vi "DSF.Engine.Framework.Create.vi"(8 "error in (no error)":errorcluster, 9 "Framework Configuration":refnum<class "DSF.Shared.Configuration.Framework.lvclass">, 10 "Framework Runtime":refnum<class "DSF.Engine.Runtime.Framework.lvclass">, 11 "Framework type":refnum<class "Framework.lvclass">) -> (0 "error out":errorcluster, 3 "Framework":refnum<class "Framework.lvclass">)   [LabVIEW 2016, in "DSF.Engine.lvlib" / "Framework.lvclass"]
uses:
  Framework.lvclass
  DSF.Engine.Runtime.Framework.lvclass
  Shared/Classes/Framework/DSF.Shared.Configuration.Framework.lvclass
  Framework.lvclass/Framework.ctl
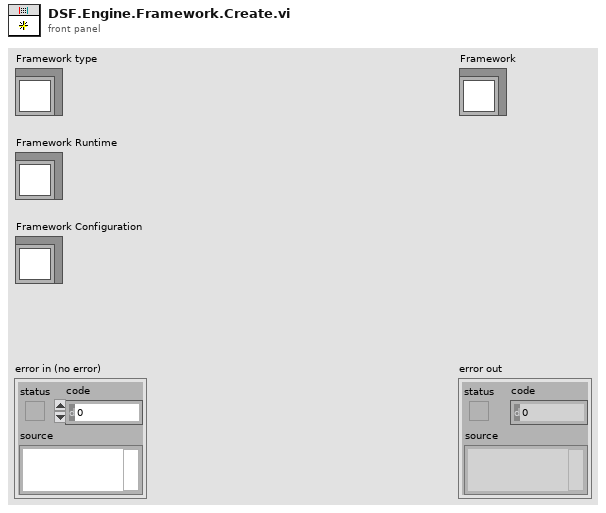
[diagram p1: front panel]
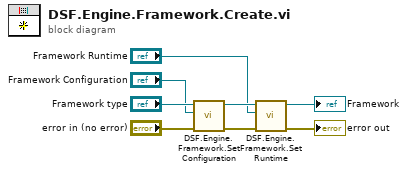
[diagram p0: block diagram]
diagram:
  n1 = call "DSF.Engine.Framework.Set Configuration.vi"("error in (no error)"="error in (no error)", "Framework Configuration"="Framework Configuration", "Framework in"="Framework type") -> ("error out"=w6:errorcluster, "Framework out"=w5:refnum<class "Framework.lvclass">)  [unwired: 7 in]
  n2 = call "DSF.Engine.Framework.Set Runtime.vi"("error in (no error)"=w6, "Framework Runtime"="Framework Runtime", "Framework in"=w5) -> ("error out"=→"error out":errorcluster, "Framework out"=→"Framework":refnum<class "Framework.lvclass">)  [unwired: 7 in]
